vi "Command & Ack - Receive Command.vi"(7 "Timeout (-1)":i32=-1, 8 "error in (no error)":errorcluster, 11 "SV B-M (Target) in":refnum<class "SV B-M (Target).lvclass">) -> (0 "error out":errorcluster, 1 "Message Data":variant, 2 "Message":string, 3 "SV B-M (Target) out":refnum<class "SV B-M (Target).lvclass">, 4 "Timeout?":bool)   [LabVIEW 2015, in "SV B-M (Target).lvclass"]
uses:
  SV B-M (Target).lvclass
  SV B-M (Target).lvclass/SV B-M (Target).ctl
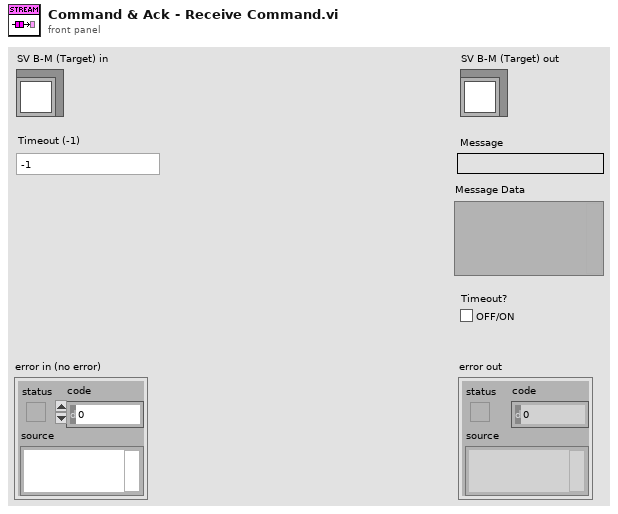
[diagram p1: front panel]
types:
  T1 = typedef "Message Cluster.ctl" = cluster{"Message":string, "Message Data":variant}
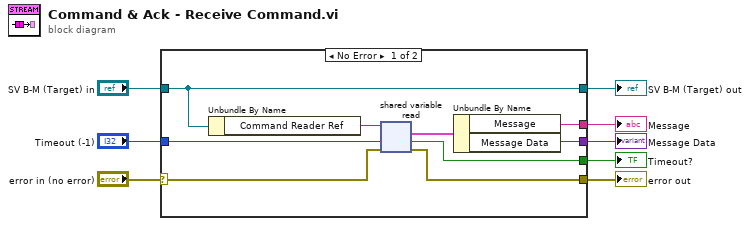
[diagram p0: block diagram]
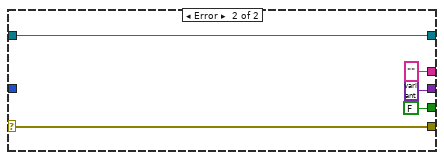
[diagram p2: hidden frame]
diagram:
  n1 = case shown="No Error" "error in (no error)" {
    selector: "error in (no error)" -> [w13 w22]
    tunnel: [w10 w22] -> w7
    tunnel: [w16 w21] -> w5
    tunnel: "SV B-M (Target) in" -> [w16 w21]
    tunnel: "Timeout (-1)" -> [w14 _]
    tunnel: [w12 "" ("Message")] -> w3
    tunnel: [w11 variant ("Message Data")] -> w2
    tunnel: [w9 FALSE] -> w1
    frame No Error {
      n2 = Unbundle By Name(w16) -> ("Command Reader Ref"=w15:refnum<k21>)
      n3 = shared-variable-read(w15, w13, w14) -> (w10:errorcluster, w9:bool, w17:T1)  [unwired: 1 out]
      n4 = Unbundle By Name(w17) -> ("Message"=w12:string, "Message Data"=w11:variant)
    }
    frame Error {
    }
  }
  "error out" <- w7
  "SV B-M (Target) out" <- w5
  "Message" <- w3
  "Message Data" <- w2
  "Timeout?" <- w1
